vi "Renishaw-XL80_SetMatCompFactor.vi"(8 "error in (no error)":errorcluster, 10 "MatCompFactor":dbl, 11 "Renishaw-XL80 in":refnum<class "Renishaw-XL80.lvclass">) -> (0 "error out":errorcluster, 3 "Renishaw-XL80 out":refnum<class "Renishaw-XL80.lvclass">)   [LabVIEW 2024, in "Renishaw-XL80.lvclass"]
doc: "Writing this property will set the material compensation factor.\n\nDefinition\nput_MatCompFactor ( [in] double newVal);\nParameters\nnewVal\nSpecifies the material compensation factor to use.\n\nComments\nThis property will return with an HRESULT of E_FAIL if the client has set AutoCompensationMode to AUTO_COMPENSATION_FULL. This warns the client that setting the material compensation factor whilst it is being automatically updated is somewhat pointless. Otherwise it will return an HRESULT of S_OK.\n\nThe material compensation factor is a factor which when multiplied by the raw laser measurement will compensate the reading for thermal growth of the material, thereby estimating the reading that would be obtained if the material temperature had been 20°C. Note that MatCompFactor is a value very close to 1.00. For example if the expansion coefficient is set to 10ppm/°C and the current material temperature is 25°C then MatCompFactor will be 0.9999"
uses:
  Renishaw-XL80.lvclass
  Renishaw-XL80.lvclass/Renishaw-XL80.ctl
  D:/A.C.M/Example CSharp_64/bin/Debug/Interop.DX10SDKADAPTORLib.dll
  Example CSharp_64/bin/Debug/Interop.DX10SDKADAPTORLib.dll
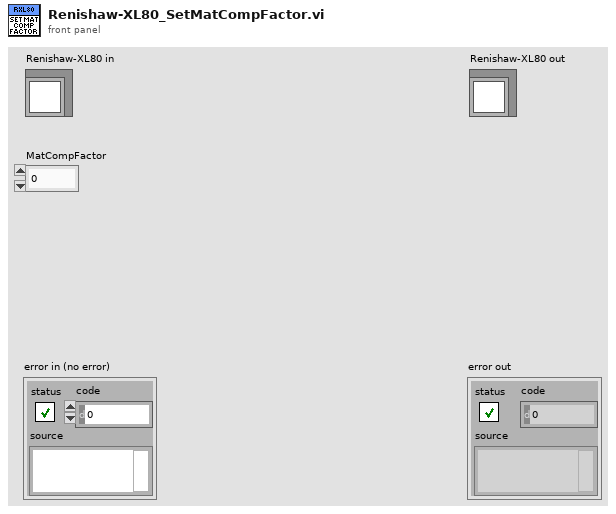
[diagram p1: front panel]
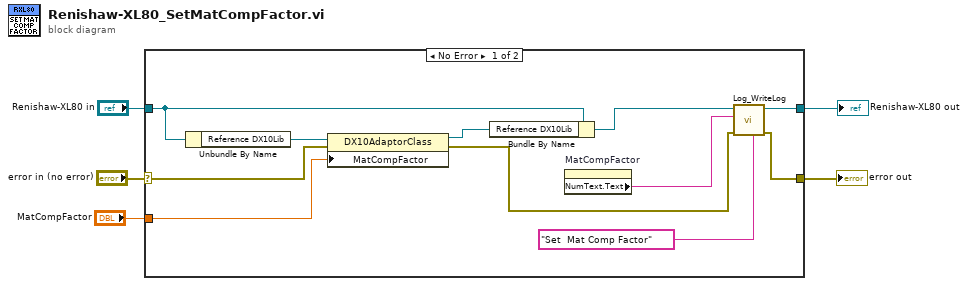
[diagram p0: block diagram]
diagram:
  n1 = case shown="No Error" "error in (no error)" {
    selector: "error in (no error)" -> [w14 w18]
    tunnel: [w7 w18] -> w4
    tunnel: [w10 w17] -> w2
    tunnel: "Renishaw-XL80 in" -> [w13 w17]
    tunnel: "MatCompFactor" -> [w12 _]
    frame No Error {
      n2 = Unbundle By Name(w13) -> ("Reference DX10Lib"=w16:refnum<k24>)
      n3 = property class="DX10AdaptorClass"(reference=w16, error in=w14, "MatCompFactor"=w12) -> (reference out=w15:refnum<k24>, error out=w6:errorcluster)
      n4 = Bundle By Name(cluster=w13, "Reference DX10Lib"=w15) -> (w11:refnum<class "Renishaw-XL80.lvclass">)
      n5 = property on="MatCompFactor" class="DigNum (strict)"() -> ("NumText.Text"=w9:string)  [unwired: 2 in, 2 out]
      n6 = call-dynamic "Log_WriteLog.vi"("Additional text"="Set  Mat Comp Factor", "error in (no error)"=w6, "Command"=w9, "Log in"=w11) -> ("error out"=w7:errorcluster, "Log out"=w10:refnum<class "Renishaw-XL80.lvclass">)  [unwired: 6 in]
    }
    frame Error {
    }
  }
  "error out" <- w4
  "Renishaw-XL80 out" <- w2
